vi "Delay_Counter.vi"() -> ()   [LabVIEW 2011]
panel:
  in  "Counter_Threshold":i32
  in  "Time_Step(ms)":i32
  in  "Delay_Count":i32
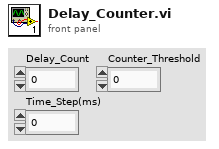
[diagram p1: front panel]
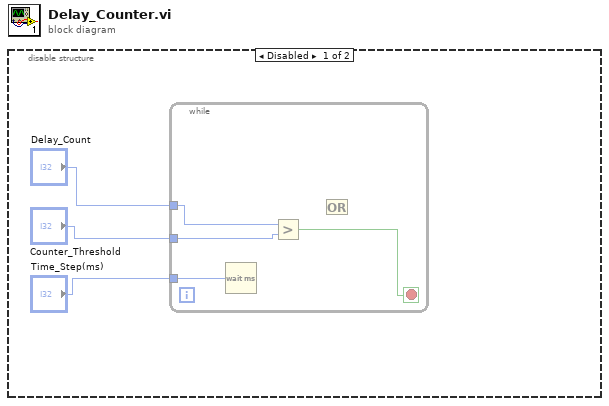
[diagram p0: block diagram]
diagram:
  n1 = disable-structure shown="Disabled" {
    frame Disabled {
      n2 = while {
        tunnel: "Delay_Count" -> [w6]
        tunnel: "Time_Step(ms)" -> [w7]
        tunnel: "Counter_Threshold" -> [w5]
        stop <- w4 stop-if-true
        n3 = Wait (ms)(milliseconds to wait=w7) -> ()  [unwired: 1 out]
        n4 = Greater?(x=w6, y=w5) -> (0:w4:bool)
        n5 = Or() -> ()  [unwired: 2 in, 1 out]
      }
    }
    frame Enabled {
    }
  }
